vi "Remove Control Panel.vi"(8 "error in (no error)":errorcluster, 10 "Process VI Name":string, 11 "Control Panels":refnum<vi>[](array[refnum])) -> (0 "error out":errorcluster)   [LabVIEW 2020]
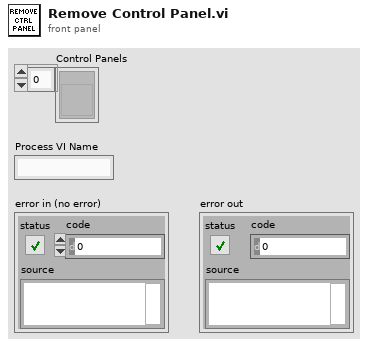
[diagram p1: front panel]
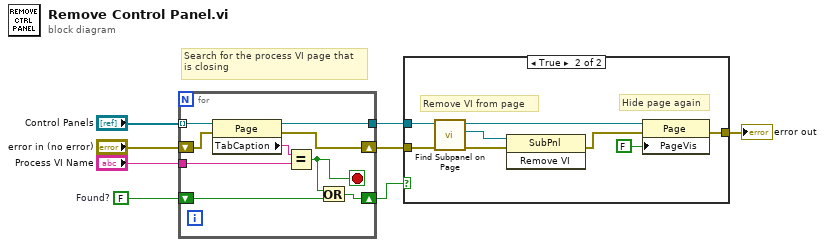
[diagram p0: block diagram]
diagram:
  w2 = FALSE  # Found?
  # "Search for the process VI page that\nis closing"
  n1 = for {
    shift-right: [w15] -> w5
    shift-left: "error in (no error)" -> [w16]
    tunnel: "Control Panels" -> [w17] mode=indexing
    tunnel: [w14] -> w6
    tunnel: "Process VI Name" -> [w12]
    shift-right: [w11] -> w1
    shift-left: w2 -> [w9]
    stop <- w10 stop-if-true
    n2 = property class="Page"(reference=w17, error in=w16) -> (reference out=w14:refnum<vi>, error out=w15:errorcluster, "TabCaption"=w13:string)
    n3 = Equal?(x=w13, y=w12) -> (x = y?=w10:bool)
    n4 = Or(x=w10, y=w9) -> (x .or. y?=w11:bool)
  }
  n5 = case shown="True" w1 {
    tunnel: [w18 w26] -> w8
    tunnel: w6 -> [_ w20]
    tunnel: w5 -> [w18 w19]
    frame False {
    }
    frame True {
      # "Remove VI from page"
      # "Hide page again"
      n6 = call "Find Subpanel on Page.vi"("error in (no error)"=w19, "Page in"=w20) -> ("error out"=w22:errorcluster, "Sub panel reference"=w21:refnum<vi>, "Page out"=w23:refnum<vi>)  [unwired: 7 in]
      n7 = invoke class="SubPnl" method="Remove VI"(reference=w21, error in=w22) -> (error out=w24:errorcluster)  [unwired: 1 in, 2 out]
      n8 = property class="Page"(reference=w23, error in=w24, "PageVis"=FALSE ("Page Visible")) -> (error out=w26:errorcluster)  [unwired: 1 out]
    }
  }
  "error out" <- w8
